vi "IP Address Harvester.vi"   [LabVIEW 2020]
uses:
  Type Definitions/Discovery Engine State.ctl
  Type Definitions/Data Frame.ctl
  Type Definitions/Data Frame Header.ctl
  Type Definitions/Payload Class.ctl
  Type Definitions/Network Adapter State.ctl
  <vilib>/Utility/tcp.llb/UDP Multicast Read-Only Open.vi
types:
  T1 = typedef "Discovery Engine State.ctl" = cluster{"Adapter IP Address":string, "Connection ID":refnum<k16>, "Error":errorcluster}
  T2 = typedef "Data Frame.ctl" = cluster{"Frame Header":T3, "Payload":string, "CRC":u32}
  T3 = typedef "Data Frame Header.ctl" = cluster{"Sync":u32, "Time":dbl, "Nanosecond Counter":i64, "Payload Class":T4, "Payload ID":u16, "Counter":u32, "Options":u32, "Source":i32, "Destination":i32}
  T4 = typedef "Payload Class.ctl" = enum16{"System State", "Parameters", "Metadata", "Software Monitor", "Data", "Commands"}
  T5 = typedef "Network Adapter State.ctl" = cluster{"Adapter IP Addresses":string[]}
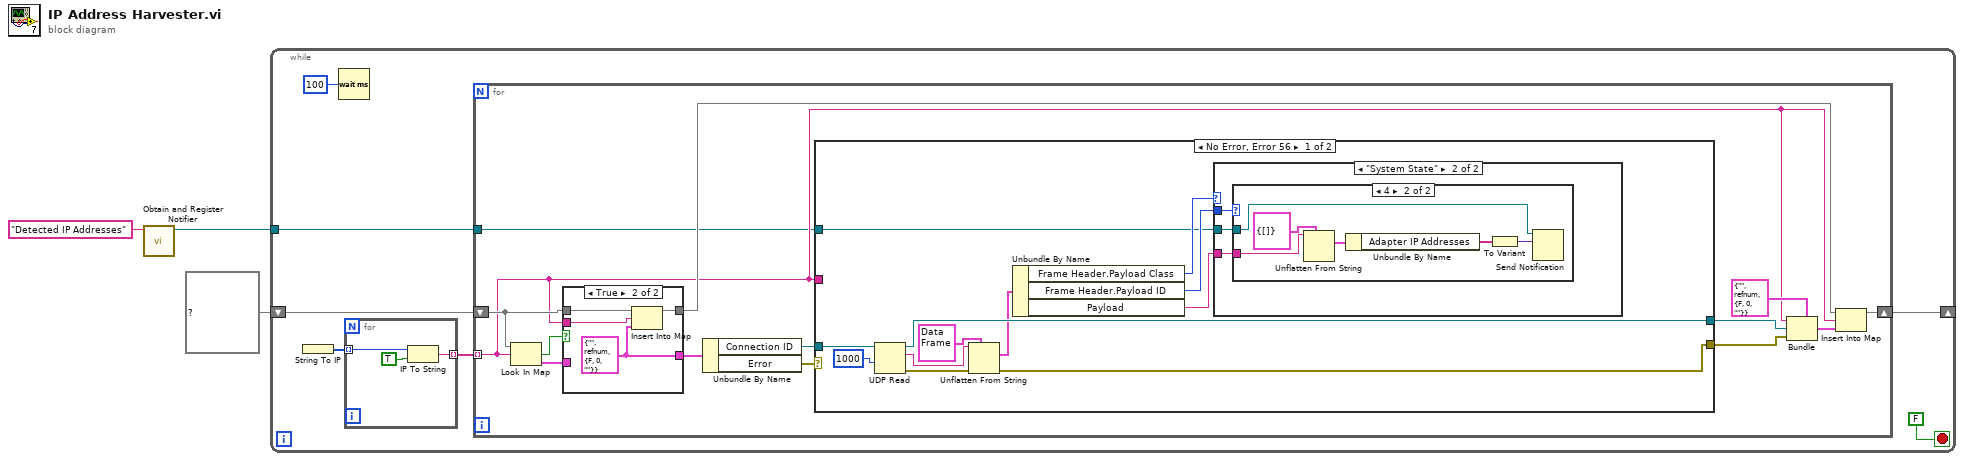
[diagram p0: block diagram]
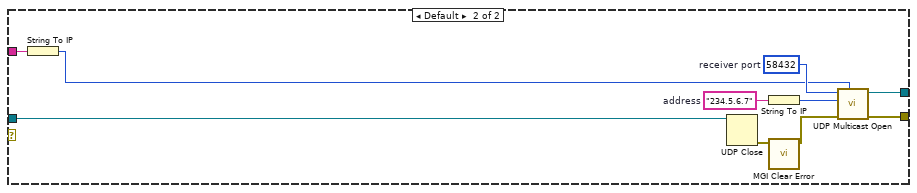
[diagram p4: hidden frame]
diagram:
  n1 = call "Obtain and Register Notifier.vi"("name (unnamed)"="Detected IP Addresses") -> ("notifier out"=w3:refnum<notifier>)  [unwired: 8 in, 2 out]
  n2 = while {
    shift-right: [w6] -> _
    shift-left: map{string, T1} {} ("map") -> [w9]
    tunnel: w3 -> [w4]
    stop <- FALSE stop-if-true
    n3 = String To IP() -> (0:w8:u32[])  [unwired: 1 in]
    n4 = Wait (ms)(milliseconds to wait=u32 100) -> ()  [unwired: 1 out]
    n5 = for {
      tunnel: w8 -> [w12] mode=indexing
      tunnel: [w11] -> w7 mode=indexing
      n6 = IP To String(1:TRUE ("dot notation? (F)"), 2:w12) -> (0:w11:string)
    }
    n7 = for {
      tunnel: w7 -> [w16] mode=indexing
      shift-right: [w15] -> w6
      shift-left: w9 -> [w26]
      tunnel: w4 -> [w14]
      n8 = Look In Map(map=w26, key=w16) -> (key not found?=w27:bool, value=w25:T1)  [unwired: 1 in]
      n9 = case shown="True" w27 {
        tunnel: w26 -> [w60 w64]
        tunnel: w16 -> [_ w63]
        tunnel: [w60 w62] -> w21
        tunnel: w25 -> [w59 _]
        tunnel: [w59 w61] -> w24
        frame False {
        }
        frame True {
          w61 = T1 {"Adapter IP Address"="", "Connection ID"=refnum, "Error"={"status"=FALSE, "code"=0, "source"=""}} ("Connection Metadata")
          n10 = Insert Into Map(map in=w64, key=w63, value=w61) -> (map out=w62:map{string, T1})  [unwired: 2 out]
        }
      }
      n11 = Unbundle By Name(w24) -> ("Connection ID"=w23:refnum<k16>, "Error"=w22:errorcluster)
      n12 = case shown="No Error, Error 56" w22 {
        tunnel: [w30 w52] -> w18
        tunnel: [w37 w51] -> w17
        tunnel: w23 -> [w38 w58]
        tunnel: w16 -> [_ w57]
        tunnel: w14 -> [w29 _]
        frame No Error {
          n13 = UDP Read(connection ID=w38, timeout ms (25000)=1000) -> (data out=w35:string, error out=w31:errorcluster, 3:w37:refnum<k16>)  [unwired: 1 in, 3 out]
          n14 = Unflatten From String(type=T2 {"Frame Header"={"Sync"=0, "Time"=0.0, "Nanosecond Counter"=0, "Payload Class"=enum."System State", "Payload ID"=0, "Counter"=0, "Options"=0, "Source"=0, "Destination"=0}, "Payload"="", "CRC"=0} ("Frame"), binary string=w35, error in (no error)=w31) -> (value=w28:T2, error out=w30:errorcluster)  [unwired: 2 in, 1 out]
          n15 = Unbundle By Name(w28) -> ("Frame Header.Payload Class"=w32:T4, "Frame Header.Payload ID"=w33:u16, "Payload"=w34:string)
          n16 = case shown="\"System State\"" w32 {
            tunnel: w34 -> [_ w42]
            tunnel: w33 -> [_ w41]
            tunnel: w29 -> [_ w40]
            frame Default {
            }
            frame "System State" {
              n17 = case shown="4" w41 {
                tunnel: w42 -> [_ w47]
                tunnel: w40 -> [_ w45]
                frame 0, Default {
                }
                frame 4 {
                  n18 = Unflatten From String(type=T5 {"Adapter IP Addresses"=[]} ("Network Adapter Metadata"), binary string=w47) -> (value=w46:T5)  [unwired: 3 in, 2 out]
                  n19 = Unbundle By Name(w46) -> ("Adapter IP Addresses"=w43:string[])
                  n20 = To Variant(anything=w43) -> (Variant=w44:variant)
                  n21 = Send Notification(notification=w44, notifier=w45) -> ()  [unwired: 1 in, 2 out]
                }
              }
            }
          }
        }
        frame Default {
          w55 = u16 58432  # receiver port
          w56 = "234.5.6.7"  # address
          n22 = String To IP(1:w57) -> (0:w53:u32)
          n23 = UDP Close(connection ID=w58) -> (error out=w50:errorcluster)  [unwired: 1 in, 1 out]
          n24 = String To IP(1:w56) -> (0:w54:u32)
          n25 = call <userlib>:"MGI Clear Error.vi"("Error In"=w50) -> ("Error Out"=w49:errorcluster)  [unwired: 6 in]
          n26 = call-poly <vilib>:"UDP Multicast Open.vi"("net address"=w53, "error in (no error)"=w49, "multicast addr"=w54, "port"=w55) -> ("error out"=w52:errorcluster, "connection ID"=w51:refnum<k16>)  [unwired: 5 in, 1 out]
        }
      }
      n27 = Bundle(cluster=T1 {"Adapter IP Address"="", "Connection ID"=refnum, "Error"={"status"=FALSE, "code"=0, "source"=""}} ("Connection Metadata"), "Adapter IP Address"=w16, "Connection ID"=w17, "Error"=w18) -> (w20:T1)
      n28 = Insert Into Map(map in=w21, key=w16, value=w20) -> (map out=w15:map{string, T1})  [unwired: 2 out]
    }
  }
